vi "configureWaveformFormat.vi"(0 "NInstrSim":refnum<class "NInstrSim.lvclass">, 2 "Waveform Format (0:ASCII)":u16(ring) items=["ASCII", "8-bit Unsigned Binary", "16-bit Signed Binary"], 3 "Byte Order (0:Low Byte First)":u16(ring) items=["Low Byte First", "High Byte First"], 5 "error in (no error)":errorcluster) -> (14 "dup NInstrSim":refnum<class "NInstrSim.lvclass">, 19 "error out":errorcluster)   [LabVIEW 2009, in "HB_Device_Examples.lvlib" / "NInstrSim.lvclass"]
doc: "Configures the format in which data is transferred from the NI Instrument Simulator.\n\nNote: Byte Order is only valid when the Waveform Format is Signed 16 bit, otherwise, the parameter is ignored."
uses:
  NInstrSim.lvclass
  lib.lib/HGF_LVC/HGF_DeviceBaseClasses/HGF_VISADevice/HGF_VISADevice.lvclass
  non_GPL/instr.lib/NI Instrument Simulator/NI Instrument Simulator.lvlib
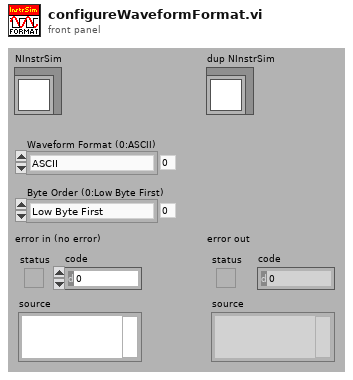
[diagram p1: front panel]
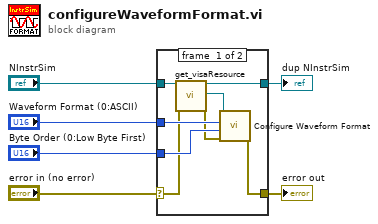
[diagram p0: block diagram]
diagram:
  n1 = case shown="No Error" "error in (no error)" {
    selector: "error in (no error)" -> [w8 w16]
    tunnel: [w7 w16] -> w5
    tunnel: [w13 w15] -> w3
    tunnel: "NInstrSim" -> [w14 w15]
    tunnel: "Waveform Format (0:ASCII)" -> [w11 _]
    tunnel: "Byte Order (0:Low Byte First)" -> [w10 _]
    frame #0 {
      n2 = call "get_visaResource.vi"("HGF_VISADevice"=w14, "error in (no error)"=w8) -> ("dup HGF_VISADevice"=w13:refnum<class "NInstrSim.lvclass">, "VISA Resource Name"=w12:refnum<visa-resource-name>, "error out"=w9:errorcluster)  [unwired: 15 out]
      n3 = call "Configure Waveform Format.vi"("error in (no error)"=w9, "Byte Order (0:Low Byte First)"=w10, "Waveform Format (0:ASCII)"=w11, "VISA resource name"=w12) -> ("error out"=w7:errorcluster)  [unwired: 7 out]
    }
    frame #1 {
    }
  }
  "error out" <- w5
  "dup NInstrSim" <- w3
